vi "list all docs.vi"() -> ()   [LabVIEW 2019]
panel:
  out "Document list":string[][](array[string])
  out "Array":string[][](array[string])
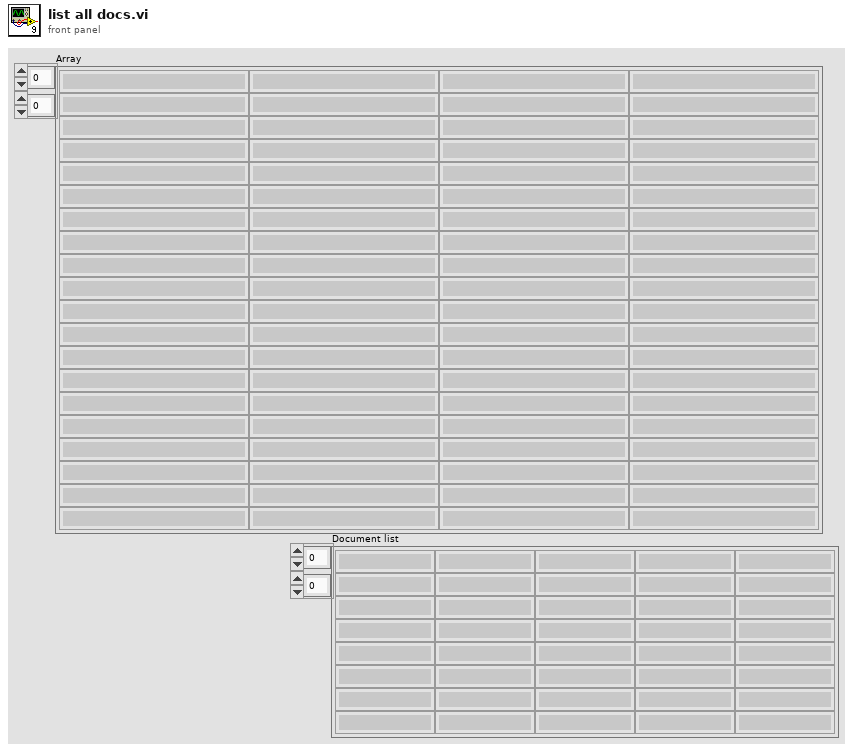
[diagram p1: front panel]
types:
  T1 = cluster{"Date":string, "On-Nonce":string, "ctype":string, "path":string, "method":string, "Authorization":string, "Accept":string, "User-Agent":string, "Content-Type":string, "secret_key":string, "access_key":string, "stack":string, "payload":string, "headers":string[], "eid":string, "wid":string, "did":string, "name":string}
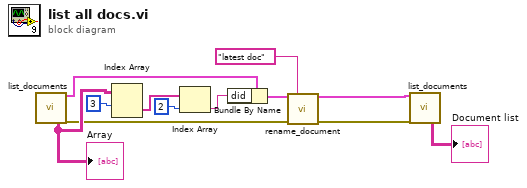
[diagram p0: block diagram]
diagram:
  n1 = call "list_documents.vi"() -> ("Document list"=w12:string[][], "Device Out"=w3:T1, "error out"=w6:errorcluster)  [unwired: 16 in, 1 out]
  "Array" <- w12
  n2 = Index Array(array=w12, index (row)=3) -> (element=w10:string[])  [unwired: 1 in]
  n3 = Index Array(array=w10, index=2) -> (element=w2:string)
  n4 = Bundle By Name(cluster=w3, "did"=w2) -> (w1:T1)
  n5 = call "rename_document.vi"("Device In"=w1, "Name"="latest doc" ("name"), "error in"=w6) -> ("Device Out"=w8:T1, "error out"=w5:errorcluster)  [unwired: 10 in, 1 out]
  n6 = call "list_documents.vi"("Device  In"=w8, "error in"=w5) -> ("Document list"=→"Document list":string[][])  [unwired: 14 in, 3 out]
